vi "E2 Data Logger.vi"(7 "refnum in":refnum<file>) -> (3 "refnum out":refnum<file>)   [LabVIEW 2014]
uses:
  <vilib>/Rock Robotics/WPI/DriverStation/WPI_DriverStationRobotMode2.ctl
  Robot Global Data.vi
  Moose Code/Auto_Conf.vi
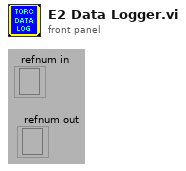
[diagram p1: front panel]
types:
  T1 = typedef "WPI_DriverStationRobotMode2.ctl" = enum16{"Autonomous Disabled", "Autonomous Enabled", "Teleop Disabled", "Teleop Enabled", "Disconnected", "Finish", "Test Disabled", "Test Enabled", "Emergency Stopped"}
  T2 = enum16{"ResetForward", "ResetBack", "PIDControl", "ManualControl", "ZeroEncoderAndTarget", "AutoStack"}
  T3 = enum16{"Disabled", "Initialize", "CalcNewTarget", "Moving", "OpenArm", "CloseArm", "Reset"}
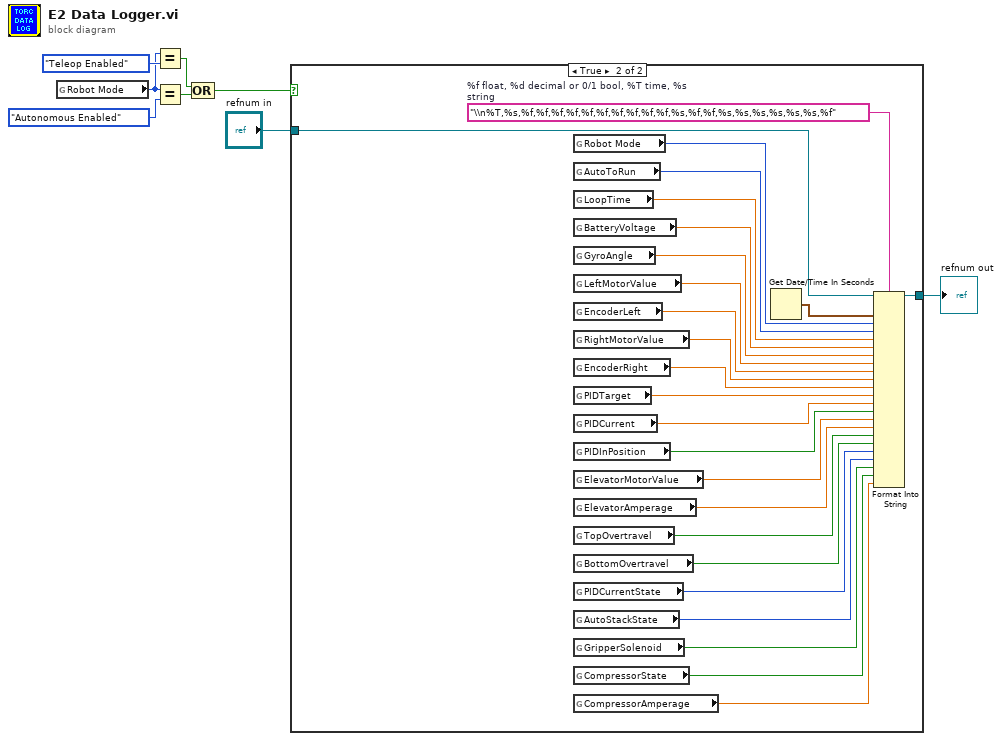
[diagram p0: block diagram]
diagram:
  n1 = global read "Robot Global Data.vi" "Robot Mode"() -> (w1:T1)
  n2 = Equal?(x=w1, y=WPI_DriverStationRobotMode2."Teleop Enabled") -> (x = y?=w4:bool)
  n3 = Equal?(x=w1, y=WPI_DriverStationRobotMode2."Autonomous Enabled") -> (x = y?=w3:bool)
  n4 = Compound Arithmetic op=OR(w4, w3) -> (w2:bool)
  n5 = case shown="True" w2 {
    tunnel: [w9 w34] -> w8
    tunnel: "refnum in" -> [w9 w10]
    frame False {
    }
    frame True {
      w31 = "\\n%T,%s,%f,%f,%f,%f,%f,%f,%f,%f,%f,%f,%s,%f,%f,%s,%s,%s,%s,%s,%s,%f"  # %f float, %d decimal or 0/1 bool, %T time, %s string
      n6 = global read "Robot Global Data.vi" "Robot Mode"() -> (w32:T1)
      n7 = global read "Auto_Conf.vi" "AutoToRun"() -> (w30:u8)
      n8 = global read "Robot Global Data.vi" "LoopTime"() -> (w29:dbl)
      n9 = global read "Robot Global Data.vi" "BatteryVoltage"() -> (w28:dbl)
      n10 = global read "Robot Global Data.vi" "GyroAngle"() -> (w27:dbl)
      n11 = global read "Robot Global Data.vi" "LeftMotorValue"() -> (w26:dbl)
      n12 = global read "Robot Global Data.vi" "EncoderLeft"() -> (w25:dbl)
      n13 = global read "Robot Global Data.vi" "RightMotorValue"() -> (w24:dbl)
      n14 = global read "Robot Global Data.vi" "EncoderRight"() -> (w23:dbl)
      n15 = global read "Robot Global Data.vi" "PIDTarget"() -> (w22:dbl)
      n16 = global read "Robot Global Data.vi" "PIDCurrent"() -> (w21:dbl)
      n17 = global read "Robot Global Data.vi" "PIDInPosition"() -> (w20:bool)
      n18 = global read "Robot Global Data.vi" "ElevatorMotorValue"() -> (w19:dbl)
      n19 = global read "Robot Global Data.vi" "ElevatorAmperage"() -> (w18:dbl)
      n20 = global read "Robot Global Data.vi" "TopOvertravel"() -> (w17:bool)
      n21 = global read "Robot Global Data.vi" "BottomOvertravel"() -> (w16:bool)
      n22 = global read "Robot Global Data.vi" "PIDCurrentState"() -> (w15:T2)
      n23 = global read "Robot Global Data.vi" "AutoStackState"() -> (w14:T3)
      n24 = global read "Robot Global Data.vi" "GripperSolenoid"() -> (w13:bool)
      n25 = global read "Robot Global Data.vi" "CompressorState"() -> (w12:bool)
      n26 = global read "Robot Global Data.vi" "CompressorAmperage"() -> (w11:dbl)
      n27 = Get Date/Time In Seconds() -> (seconds since 1Jan1904=w33:timestamp)
      n28 = Format Into String(format string=w31, initial string=w10, w33, w32, w30, w29, w28, w27, w26, w25, w24, w23, w22, w21, w20, w19, w18, w17, w16, w15, w14, w13, w12, w11) -> (resulting string=w34:refnum<file>)  [unwired: 1 in, 1 out]
    }
  }
  "refnum out" <- w8
